vi "CRITICAL.vi"(6 "Message":string, 8 "error in":errorcluster) -> (0 "error out":errorcluster)   [LabVIEW 2020, in "hse-logger.lvlib"]
doc: "Logs a message and the content of the error-cluster, if \"error in\" is True.\nAn error on the \"error in\" terminal is cleared on the \"error out\" terminal.\n\n____\nHAMPEL SOFTWARE ENGINEERING v2.0.6 (2021-04-15 11:38)"
uses:
  hse-logger.lvlib
  Logger/Logger.lvclass
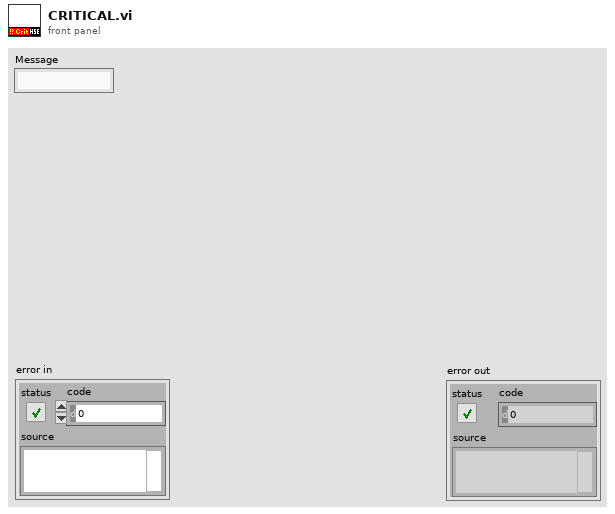
[diagram p1: front panel]
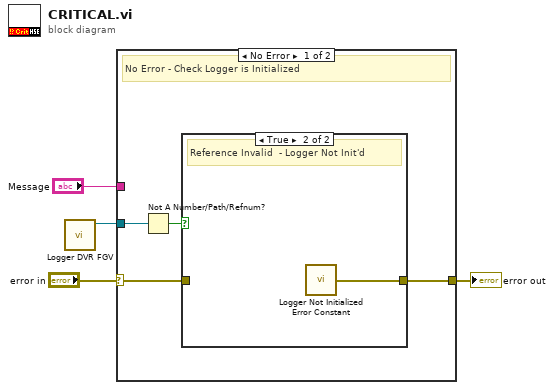
[diagram p0: block diagram]
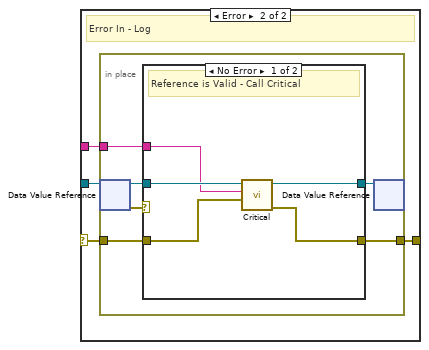
[diagram p3: hidden frame]
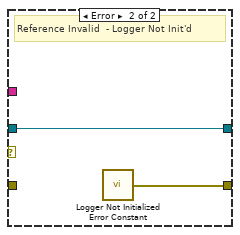
[diagram p4: hidden frame]
diagram:
  n1 = call "Logger DVR FGV.vi"() -> ("Logger DVR"=w2:refnum<data-value>)  [unwired: 10 in, 1 out]
  n2 = case shown="No Error" "error in" {
    selector: "error in" -> [w6 w12]
    tunnel: "Message" -> [_ w14]
    tunnel: [w5 w13] -> w3
    tunnel: w2 -> [w8 w11]
    frame No Error {
      # "No Error - Check Logger is Initialized"
      n3 = Not A Number/Path/Refnum?(number/path/refnum=w8) -> (NaN/Path/Refnum?=w7:bool)
      n4 = case shown="True" w7 {
        tunnel: w6 -> [w9 _]
        tunnel: [w9 w10] -> w5
        frame False {
          # "Reference is Valid - Do Nothing"
        }
        frame True {
          # "Reference Invalid  - Logger Not Init'd"
          n5 = call "Logger Not Initialized Error Constant.vi"() -> ("Logger Not Initialized Error"=w10:errorcluster)
        }
      }
    }
    frame Error {
      # "Error In - Log"
      n6 = in-place {
        in-place-border: w14 -> [w19]
        in-place-border: [w18] -> w13
        in-place-border: w12 -> [w15]
        n7 = in-place-dvr #1(w11) -> (w20:refnum<class "Logger.lvclass">, w16:errorcluster)
        n8 = case shown="No Error" w16 {
          tunnel: w20 -> [w25 w27]
          tunnel: w19 -> [w24 _]
          tunnel: [w23 w26] -> w18
          tunnel: [w22 w27] -> w17
          tunnel: w15 -> [w21 _]
          frame No Error {
            # "Reference is Valid - Call Critical"
            n9 = call-dynamic "Critical.vi"("Error to Log"=w21, "Message"=w24, "Logger in"=w25) -> ("error out"=w23:errorcluster, "Logger out"=w22:refnum<class "Logger.lvclass">)  [unwired: 7 in]
          }
          frame Error {
            # "Reference Invalid  - Logger Not Init'd"
            n10 = call "Logger Not Initialized Error Constant.vi"() -> ("Logger Not Initialized Error"=w26:errorcluster)
          }
        }
        n11 = in-place-dvr #1(w17) -> ()  [unwired: 2 out]
      }
    }
  }
  "error out" <- w3
